vi "obtener productos.vi"(8 "error in (no error)":errorcluster, 10 "Productos":T1) -> (0 "error out":errorcluster)   [LabVIEW 2020, in "Configuracion.lvlib"]
doc: "Obtains the products actualization from the Config Module\n_____\nCreated using Delacor QMH Event Scripter 5.0.0.112."
uses:
  Configuracion.lvlib
  obtener productos Argument--cluster.ctl
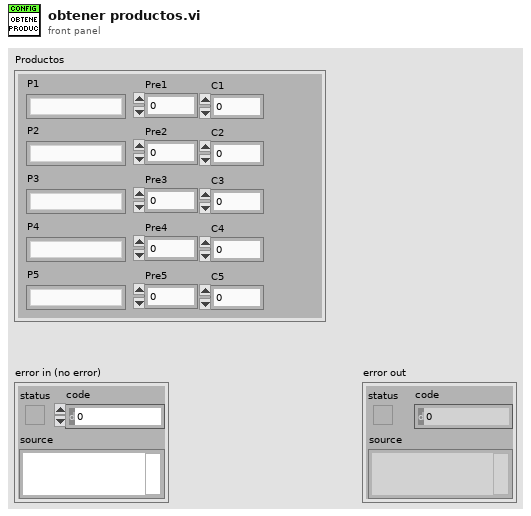
[diagram p1: front panel]
types:
  T1 = cluster{"P1":string, "Pre1":dbl, "C1":dbl, "P2":string, "Pre2":dbl, "C2":dbl, "P3":string, "Pre3":dbl, "C3":dbl, "P4":string, "Pre4":dbl, "C4":dbl, "P5":string, "Pre5":dbl, "C5":dbl}
  T2 = typedef "Configuracion.lvlib/obtener productos Argument--cluster.ctl" = cluster{"Productos":cluster{"P1":string, "Pre1":dbl, "C1":dbl, "P2":string, "Pre2":dbl, "C2":dbl, "P3":string, "Pre3":dbl, "C3":dbl, "P4":string, "Pre4":dbl, "C4":dbl, "P5":string, "Pre5":dbl, "C5":dbl}}
  T3 = typedef "Configuracion.lvlib/Request Events--cluster.ctl" = cluster{"Stop Module":refnum<user-event>, "Show Panel":refnum<user-event>, "Hide Panel":refnum<user-event>, "Get Module Execution Status":refnum<user-event>, "Show Diagram":refnum<user-event>, "obtener productos":refnum<user-event>}
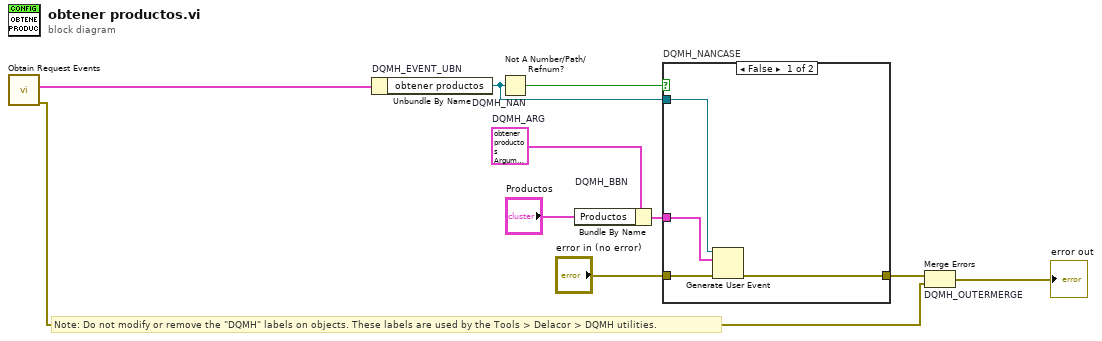
[diagram p0: block diagram]
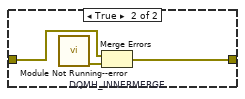
[diagram p2: hidden frame]
diagram:
  w4 = T2 {"Productos"={"P1"="", "Pre1"=0.0, "C1"=0.0, "P2"="", "Pre2"=0.0, "C2"=0.0, "P3"="", "Pre3"=0.0, "C3"=0.0, "P4"="", "Pre4"=0.0, "C4"=0.0, "P5"="", "Pre5"=0.0, "C5"=0.0}}  # DQMH_ARG
  # "Note: Do not modify or remove the \"DQMH\" labels on objects. These labels are used by the Tools > Delacor > DQMH utilities."
  n1 = call "Obtain Request Events.vi"() -> ("error out"=w2:errorcluster, "Configuracion Request Events"=w1:T3)  [unwired: 10 in]
  n2 = Unbundle By Name "DQMH_EVENT_UBN"(w1) -> ("obtener productos"=w6:refnum<user-event>)
  n3 = Not A Number/Path/Refnum? "DQMH_NAN"(number/path/refnum=w6) -> (NaN/Path/Refnum?=w7:bool)
  n4 = Bundle By Name "DQMH_BBN"(cluster=w4, "Productos"="Productos") -> (w8:T2)
  n5 = case "DQMH_NANCASE" shown="False" w7 {
    tunnel: "error in (no error)" -> [w14 w17]
    tunnel: [w13 w16] -> w5
    tunnel: w6 -> [w12 _]
    tunnel: w8 -> [w11 _]
    frame False {
      n6 = Generate User Event(user event=w12, event data cluster=w11, error in=w14) -> (error out=w13:errorcluster)  [unwired: 1 in, 1 out]
    }
    frame True {
      n7 = call "Module Not Running--error.vi"() -> ("error out"=w15:errorcluster)  [unwired: 11 in]
      n8 = Merge Errors "DQMH_INNERMERGE"(w17, w15) -> (w16:errorcluster)
    }
  }
  n9 = Merge Errors "DQMH_OUTERMERGE"(w5, w2) -> (→"error out":errorcluster)
